vi "Get PPL Version Number.vi"(8 "Error In":errorcluster, 11 "EXE Filepath":path) -> (0 "Error Out":errorcluster, 3 "PPL Version Number":string)   [LabVIEW 2023, in "Error Manager.lvlib"]
doc: "Retrieves the File Version of an EXE."
uses:
  Error Manager.lvlib
panel:
  # "Development\ncontrols/indicators useful for development and testing, but which are not outputs of the VI"
  # "Input\nInputs to the VI"
  # "Output\nOutputs of the VI"
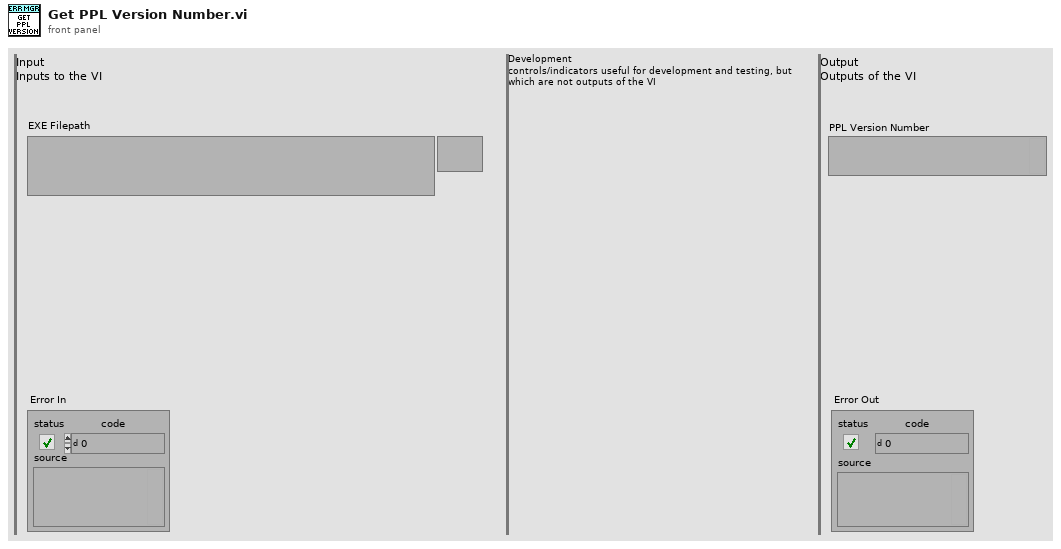
[diagram p1: front panel]
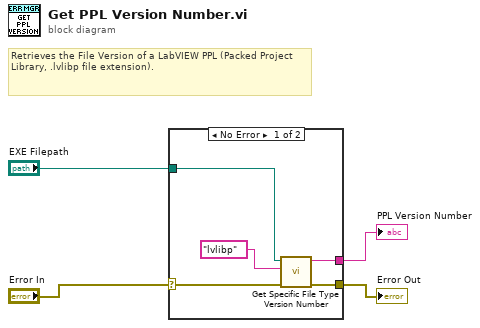
[diagram p0: block diagram]
diagram:
  # "Retrieves the File Version of a LabVIEW PPL (Packed Project Library, .lvlibp file extension)."
  n1 = case shown="No Error" "Error In" {
    selector: "Error In" -> [w7 w10]
    tunnel: [w6 w10] -> w3
    tunnel: "EXE Filepath" -> [w9 _]
    tunnel: [w5 _] -> w1
    frame No Error {
      n2 = call "Get Specific File Type Version Number.vi"("error in"=w7, "Specific File Extension (e.g \"exe\", \"dll\" or \"lvlibp\")"="lvlibp" ("expected file extension (e.g \"txt\")"), "Filepath"=w9) -> ("error out"=w6:errorcluster, "File Version Number"=w5:string)  [unwired: 7 in]
    }
    frame Error {
    }
  }
  "Error Out" <- w3
  "PPL Version Number" <- w1
